vi "PSVCH_Caculate Thread.vi"() -> ()   [LabVIEW 2016]
uses:
  SubVIs/State.ctl
  ToolKit/Formula/Ctrls/PSFormula_FOR_Formula Node.ctl
  ToolKit/Formula/Ctrls/PSFormula_FOR_Formula Step.ctl
  ToolKit/Formula/Ctrls/PSFormula_FOR_Formula Para.ctl
  ToolKit/Formula/Ctrls/PSFormula_FOR_Formula MidVar Data.ctl
  Ctrls/PSVCH_VarList.ctl
  <vilib>/Platform/TimedLoop/XDataNode/timing_clust.ctl
  <vilib>/Platform/TimedLoop/XDataNode/nitl_modes.ctl
  <vilib>/Platform/TimedLoop/XDataNode/wakeup.ctl
  <vilib>/Platform/TimedLoop/TimeConversion.llb/rt-timestamp-to-milliseconds.vi
  Architecture/Queue Management/ARC_Queue Insert Element.vi
  <vilib>/Platform/TimedLoop/XDataNode/XDataNode.xnode
  <vilib>/Platform/TimedLoop/XDataNode/XDNodeRunTimeDep.lvlib
  <vilib>/measure/NI_MABase.lvlib
panel:
  in  "State":T1
  in  "Parameter":variant
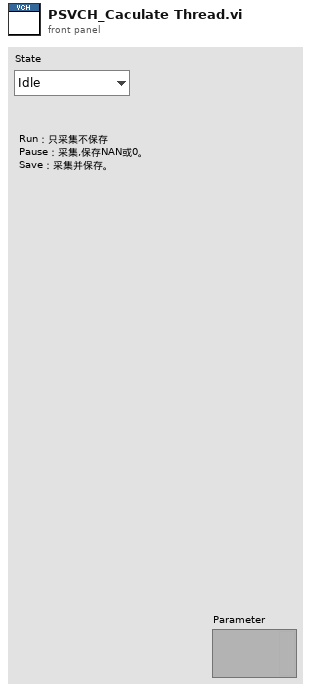
[diagram p1: front panel]
types:
  T1 = typedef "State.ctl" = enum16{"Idle", "Run", "Pause", "Save"}
  T2 = typedef "PSFormula_FOR_Formula Node.ctl" = cluster{"Formula Steps":T3[], "MidVar List":T5}
  T3 = typedef "PSFormula_FOR_Formula Step.ctl" = cluster{"Formula Calc":string, "Para":T4[], "Result Var":string, "Result Var Type":string}
  T4 = typedef "PSFormula_FOR_Formula Para.ctl" = cluster{"Para Index":i32, "Tag":string, "Type":string, "Label":string, "Data":variant}
  T5 = typedef "PSFormula_FOR_Formula MidVar Data.ctl" = cluster{"Names":string[], "Types":string[], "Values":variant[]}
  T6 = typedef "PSVCH_VarList.ctl" = cluster{"Tag[]":string[], "Type[]":string[], "Value[]":variant[], "ai[]":string[]}
  T7 = cluster{"Q_High Name":string, "Tag":string, "t0":timestamp, "Period":i64, "Exit":refnum<notifier>, "Dpl":refnum<queue>, "TDMS Ref":refnum<notifier>, "Save":refnum<notifier>, "Formula Node 2":T2, "VarList":T6, "Save?":bool, "Name":string, "Unit":string}
  T8 = typedef "XDNodeRunTimeDep.lvlib/timing_clust.ctl" = cluster{"Expected End [f-1]":u64, "Actual End [f-1]":u64, "Finished Late? [f-1]":bool, "Expected End [i-1]":u64, "Actual End [i-1]":u64, "Finished Late? [i-1]":bool, "Expected Start [i]":u64, "Actual Start [i]":u64, "Expected Start [f]":u64, "Actual Start [f]":u64, "Source Name":string, "Structure Name":string, "Period":i64, "Deadline":i64, "Offset":i64, "Start":i64, "Priority":i32, "Timeout":i32, "Mode":T9, "Wakeup Reason":T10, "Error":errorcluster, "Source Type":string, "Secondary Source Type":string, "Global End Time":u64, "Global Start Time":u64, "Frame Duration":u64, "Iteration Duration":u64, "Assigned CPU":i32, "I/O Scan Engine Mode":u32}
  T9 = typedef "XDNodeRunTimeDep.lvlib/nitl_modes.ctl" = enum32{"No Change", "Process missed periods, maintain original phase", "Discard missed periods, maintain original phase", "Process missed periods, ignore original phase", "Discard missed periods, ignore original phase"}
  T10 = typedef "XDNodeRunTimeDep.lvlib/wakeup.ctl" = enum32{"Normal", "Aborted", "Asynchronous wakeup", "Timing source error", "Timed loop error", "Timeout"}
  T11 = cluster{"ai[]":string[], "Type[]":string[], "Value[]":variant[]}
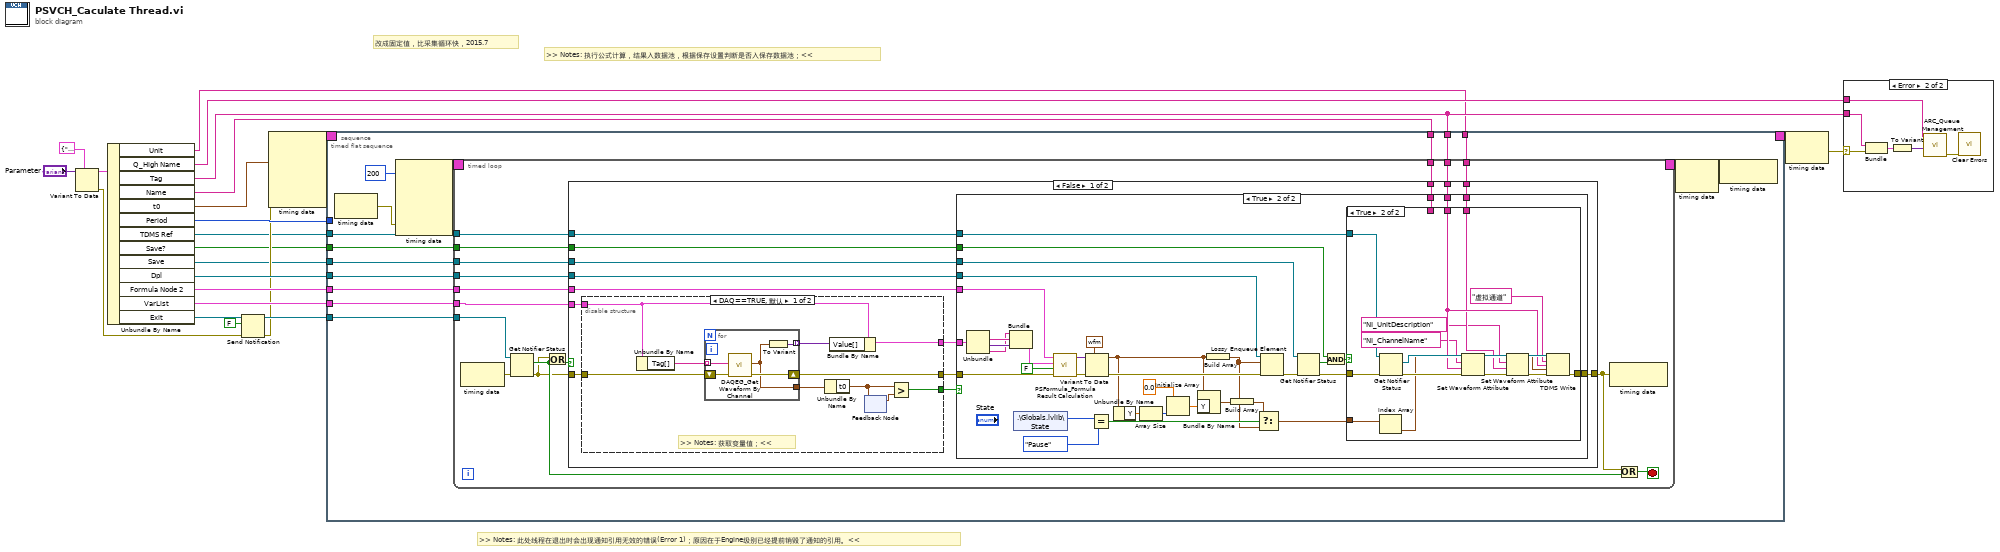
[diagram p0: block diagram]
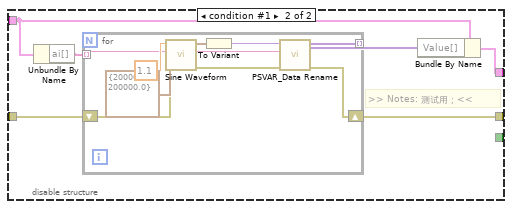
[diagram p4: hidden frame]
diagram:
  # "改成固定值，比采集循环快，2015.7"
  # ">> Notes: 此处线程在退出时会出现通知引用无效的错误(Error 1)；原因在于Engine级别已经提前销毁了通知的引用。<<"
  # ">> Notes: 执行公式计算，结果入数据池，根据保存设置判断是否入保存数据池；<<"
  n1 = Variant To Data(type=T7 {"Q_High Name"="", "Tag"="", "t0"=timestamp(0 s since 1904-01-01), "Period"=0, "Exit"=refnum, "Dpl"=refnum, "TDMS Ref"=refnum, "Save"=refnum, "Formula Node 2"={"Formula Steps"=[], "MidVar List"={"Names"=[], "Types"=[], "Values"=[]}}, "VarList"={"Tag[]"=[], "Type[]"=[], "Value[]"=[], "ai[]"=[]}, "Save?"=FALSE, "Name"="", "Unit"=""} ("Para"), Variant="Parameter") -> (data=w23:T7, error out=w10:errorcluster)  [unwired: 1 in]
  n2 = Unbundle By Name(w23) -> ("Unit"=w1:string, "Q_High Name"=w21:string, "Tag"=w5:string, "Name"=w3:string, "t0"=w13:timestamp, "Period"=w14:i64, "TDMS Ref"=w7:refnum<notifier>, "Save?"=w4:bool, "Save"=w6:refnum<notifier>, "Dpl"=w20:refnum<queue>, "Formula Node 2"=w19:T2, "VarList"=w18:T6, "Exit"=w12:refnum<notifier>)
  n3 = Send Notification(notification=FALSE ("通知"), notifier=w12, error in (no error)=w10) -> (notifier out=w11:refnum<notifier>, error out=w8:errorcluster)
  n4 = node-c288(w13, w8) -> (w17:T8)  [unwired: 3 in]
  n5 = timed-sequence {
    timing: w17 -> [_]
    timing-out: [_] -> w16
    tunnel: w14 -> [w34]
    tunnel: w20 -> [w33]
    tunnel: w19 -> [w32]
    tunnel: w18 -> [w31]
    tunnel: w11 -> [w30]
    tunnel: w7 -> [w29]
    tunnel: w6 -> [w28]
    tunnel: w5 -> [w27]
    tunnel: w4 -> [w26]
    tunnel: w3 -> [w25]
    tunnel: w1 -> [w24]
    n6 = timed-flat-sequence {
      tunnel: w34 -> [_]
      tunnel: w33 -> [w47]
      tunnel: w32 -> [w46]
      tunnel: w31 -> [w45]
      tunnel: w30 -> [w43]
      tunnel: w29 -> [w41]
      tunnel: w28 -> [w40]
      tunnel: w27 -> [w39]
      tunnel: w26 -> [w38]
      tunnel: w25 -> [w37]
      tunnel: w24 -> [w36]
      n7 = node-c288() -> (w42:errorcluster)  [unwired: 1 in]
      n8 = node-c288(i64 200 ("周期"), w42) -> (w49:T8)  [unwired: 3 in]
      n9 = timed-loop {
        timing: w49 -> [_]
        timing-out: [_] -> w48
        tunnel: w47 -> [w63]
        tunnel: w46 -> [w65]
        tunnel: w45 -> [w64]
        tunnel: w43 -> [w61]
        tunnel: w41 -> [w56]
        tunnel: w40 -> [w57]
        tunnel: w39 -> [w55]
        tunnel: w38 -> [w54]
        tunnel: w37 -> [w53]
        tunnel: w36 -> [w50]
        stop <- w58 stop-if-true
        n10 = node-c288() -> (w62:errorcluster)  [unwired: 1 in]
        n11 = Get Notifier Status(notifier=w61, error in (no error)=w62) -> (current notification=w59:bool, error out=w51:errorcluster)  [unwired: 3 out]
        n12 = Or(x=w51, y=w59) -> (x .or. y?=w52:bool)
        n13 = case shown="False" w52 {
          tunnel: w65 -> [w70 _]
          tunnel: w64 -> [w79 _]
          tunnel: [w75 w164] -> w60
          tunnel: w63 -> [w78 _]
          tunnel: w51 -> [w77 w164]
          tunnel: w57 -> [w76 _]
          tunnel: w56 -> [w74 _]
          tunnel: w55 -> [w73 _]
          tunnel: w54 -> [w72 _]
          tunnel: w53 -> [w71 _]
          tunnel: w50 -> [w67 _]
          frame False {
            n14 = disable-structure shown="DAQ==TRUE, 默认" {
              disable-tunnel: w79 -> [w143 w151]
              disable-tunnel: [w142 w154] -> w69
              disable-tunnel: w77 -> [w139 w153]
              disable-tunnel: [w138 w152] -> w68
              disable-tunnel: [w134 _] -> w66
              frame condition #0 (active) {
                # ">> Notes: 获取变量值；<<"
                n15 = Unbundle By Name(w143) -> ("Tag[]"=w140:string[])
                n16 = for {
                  tunnel: [w148] -> w141 mode=indexing
                  tunnel: w140 -> [w145] mode=indexing
                  shift-right: [w146] -> w138
                  shift-left: w139 -> [w147]
                  tunnel: [w144] -> w135
                  n17 = call "DAQEG_Get Waveform By Channel.vi"("error in"=w147, "DAQ Channel"=w145) -> ("error out"=w146:errorcluster, "waveform"=w144:waveform(dbl))  [unwired: 8 in]
                  n18 = To Variant(anything=w144) -> (Variant=w148:variant)
                }
                n19 = Unbundle By Name(w135) -> ("t0"=w136:timestamp)
                n20 = Bundle By Name(cluster=w143, "Value[]"=w141) -> (w142:T6)
                n21 = feedback #1() -> (w137:timestamp)  [unwired: 1 in]
                n22 = feedback-in #1(w136) -> ()
                n23 = Greater?(x=w136, y=w137) -> (0:w134:bool)
              }
              frame condition #1 {
                # ">> Notes: 测试用；<<"
                n24 = Unbundle By Name(w151) -> ("ai[]"=w150:string[])
                n25 = for {
                  tunnel: [w158] -> w149 mode=indexing
                  tunnel: w150 -> [w155] mode=indexing
                  shift-right: [w156] -> w152
                  shift-left: w153 -> [w160]
                  n26 = call <vilib>:"Sine Waveform.vi"("sampling info"=cluster{"Fs":dbl, "#s":dbl} {"Fs"=200000.0, "#s"=200000.0}, "error in (no error)"=w160, "frequency"=1.1) -> ("error out"=w157:errorcluster, "signal out"=w161:waveform(dbl))  [unwired: 7 in]
                  n27 = To Variant(anything=w161) -> (Variant=w159:variant)
                  n28 = call "PSVAR_Data Rename.vi"("error in"=w157, "Name New"=w155, "Data In"=w159) -> ("error out"=w156:errorcluster, "Data Out"=w158:variant)  [unwired: 7 in]
                }
                n29 = Bundle By Name(cluster=w151, "Value[]"=w149) -> (w154:T6)
              }
            }
            n30 = case shown="True" w66 {
              tunnel: w78 -> [_ w116]
              tunnel: w76 -> [_ w114]
              tunnel: [w80 w112] -> w75
              tunnel: w74 -> [_ w111]
              tunnel: w73 -> [_ w110]
              tunnel: w72 -> [_ w108]
              tunnel: w71 -> [_ w106]
              tunnel: w70 -> [_ w105]
              tunnel: w69 -> [_ w104]
              tunnel: w68 -> [w80 w97]
              tunnel: w67 -> [_ w93]
              frame False {
              }
              frame True {
                n31 = Unbundle(w104) -> ("Type[]"=w103:string[], "Value[]"=w102:variant[], "ai[]"=w98:string[])  [unwired: 1 out]
                n32 = Bundle("ai[]"=w98, "Type[]"=w103, "Value[]"=w102) -> (w101:T11)  [unwired: 1 in]
                n33 = shared-variable ".\\Globals.lvlib\\State"() -> (w92:T1)  [unwired: 1 in, 1 out]
                n34 = call "PSFormula_Formula Result Calculation.vi"("error in"=w97, "Complex Variable(T)"=FALSE, "Var List"=w101, "Formula Node"=w105) -> ("error out"=w96:errorcluster, "Result Value"=w100:variant)  [unwired: 5 in, 1 out]
                n35 = Variant To Data(error in=w96, type=waveform(dbl) {"t0"=timestamp(0 s since 1904-01-01), "dt"=1.0, "Y"=[]} ("Waveform"), Variant=w100) -> (data=w88:waveform(dbl), error out=w95:errorcluster)
                n36 = Equal?(x=w92, y=State."Pause") -> (x = y?=w90:bool)
                n37 = Unbundle By Name(w88) -> ("Y"=w87:dbl[])
                n38 = Array Size(array=w87) -> (size(s)=w85:i32)
                n39 = Initialize Array(0.0 ("元素"), w85) -> (w86:dbl[])
                n40 = Bundle By Name(cluster=w88, "Y"=w86) -> (w83:waveform(dbl))
                n41 = Build Array(w88) -> (w89:waveform(dbl)[])
                n42 = Build Array(w83) -> (w82:waveform(dbl)[])
                n43 = Select(t=w82, s=w90, f=w89) -> (s? t:f=w81:waveform(dbl)[])
                n44 = Lossy Enqueue Element(queue=w116, element=w89, error in (no error)=w95) -> (error out=w115:errorcluster)  [unwired: 3 out]
                n45 = Get Notifier Status(notifier=w114, error in (no error)=w115) -> (current notification=w109:bool, error out=w113:errorcluster)  [unwired: 3 out]
                n46 = And(x=w108, y=w109) -> (x .and. y?=w107:bool)
                n47 = case shown="True" w107 {
                  tunnel: w113 -> [w117 w133]
                  tunnel: [w117 w130] -> w112
                  tunnel: w111 -> [_ w132]
                  tunnel: w81 -> [_ w128]
                  tunnel: w110 -> [_ w125]
                  tunnel: w106 -> [_ _]
                  tunnel: w93 -> [_ w119]
                  frame False {
                  }
                  frame True {
                    n48 = Index Array(array=w128) -> (element=w126:waveform(dbl))  [unwired: 1 in]
                    n49 = Get Notifier Status(notifier=w132, error in (no error)=w133) -> (current notification=w131:refnum<k34>, error out=w127:errorcluster)  [unwired: 3 out]
                    n50 = Set Waveform Attribute(4:w127, 5:w125, 6:"NI_ChannelName" ("名称"), 7:w126) -> (0:w123:errorcluster, 3:w121:waveform(dbl))  [unwired: 1 out]
                    n51 = Set Waveform Attribute(4:w123, 5:w119, 6:"NI_UnitDescription" ("名称"), 7:w121) -> (0:w122:errorcluster, 3:w120:waveform(dbl))  [unwired: 1 out]
                    n52 = TDMS Write(0:w131, 5:"虚拟通道" ("组名称输入（无标题）"), 7:w125, 9:w120, 11:w122) -> (15:w130:errorcluster)  [unwired: 1 in, 3 out]
                  }
                }
              }
            }
          }
          frame True {
          }
        }
        n53 = node-c288(w60) -> ()  [unwired: 1 out]
        n54 = Or(x=w60, y=w59) -> (x .or. y?=w58:bool)
      }
      n55 = node-c288(w48) -> (w44:errorcluster)
      n56 = node-c288(w44) -> ()  [unwired: 1 out]
    }
  }
  n57 = node-c288(w16) -> (w15:errorcluster)
  n58 = case shown="Error" w15 {
    selector: w15 -> [_ w185]
    tunnel: w21 -> [_ w183]
    tunnel: w5 -> [_ w181]
    frame No Error {
    }
    frame Error {
      n59 = Bundle("Tag"=w181, "error IO"=w185) -> (w184:cluster{"Tag":string, "error IO":errorcluster})  [unwired: 1 in]
      n60 = To Variant(anything=w184) -> (Variant=w186:variant)
      n61 = call-poly "ARC_Queue Management.vi"("Data"=w186, "Queue Name(unamed)"=w183) -> ("error out"=w182:errorcluster)  [unwired: 8 in, 1 out]
      n62 = call <vilib>:"Clear Errors.vi"("error in (no error)"=w182) -> ()  [unwired: 5 in, 2 out]
    }
  }
